vi "RangeGlobal_FLo.vi"() -> ()   [LabVIEW 2013]
panel:
  out "RangeGlobal":u8[](array[numeric])
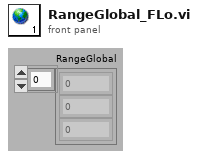
[diagram p1: front panel]
diagram:
